vi "Serial Number Read-Write, standalone.vi"() -> ()   [LabVIEW 2015]
panel:
  out "Serial Number returned":u16 format="%04x"
  in  "Serial Number":u16
  out "ACK ok":bool
  in  "VISA resource name in":refnum<visa-resource-name>
  out "Error out":errorcluster
  in  "R / W":string(combo)="R"
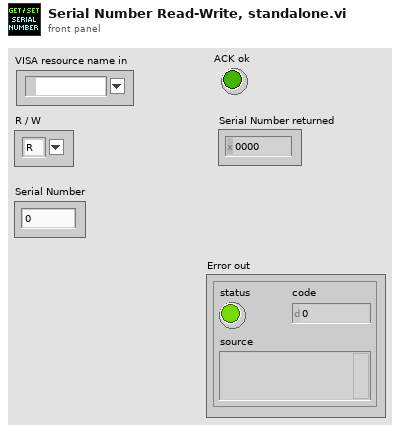
[diagram p1: front panel]
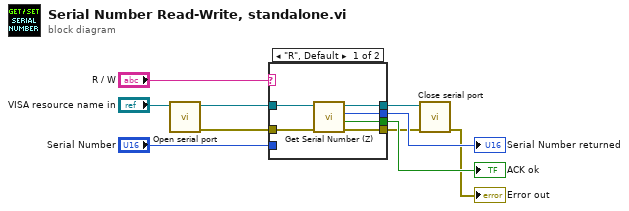
[diagram p0: block diagram]
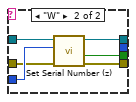
[diagram p2: hidden frame]
diagram:
  n1 = call "Open serial port.vi"("VISA resource name"="VISA resource name in") -> ("Error out"=w1:errorcluster, "VISA resource name out"=w7:refnum<visa-resource-name>)  [unwired: 9 in]
  n2 = case shown="\"R\", Default" "R / W" {
    tunnel: "Serial Number" -> [_ w22]
    tunnel: w7 -> [w16 w21]
    tunnel: [w15 w19] -> w3
    tunnel: [w14 _] -> w6
    tunnel: [w13 w18] -> w5
    tunnel: [w12 w20] -> w4
    tunnel: w1 -> [w11 w17]
    frame "R", Default {
      n3 = call "Get Serial Number (Z).vi"("VISA resource name in"=w16, "Error In"=w11) -> ("VISA resource name out"=w12:refnum<visa-resource-name>, "Serial Number"=w14:u16, "ACK"=w13:bool, "Error out"=w15:errorcluster)  [unwired: 5 in]
    }
    frame "W" {
      n4 = call "Set Serial Number (z).vi"("Error In"=w17, "Serial Number"=w22, "VISA resource name in"=w21) -> ("Error out"=w19:errorcluster, "ACK"=w18:bool, "VISA resource name out"=w20:refnum<visa-resource-name>)  [unwired: 6 in]
    }
  }
  "ACK ok" <- w5
  "Serial Number returned" <- w6
  n5 = call "Close serial port.vi"("Error in"=w3, "VISA resource name"=w4) -> ("Error out"=→"Error out":errorcluster)  [unwired: 9 in]
